vi "ApplyTableBlockAppearance.vi"(5 "Check Mode?":bool, 6 "changed? subarray":bool[][](array[boolean]), 7 "Change start":T1, 8 "error in (no error)":errorcluster, 9 "Mode Index":i32=2, 10 "Col Array in":refnum<class "Column.lvclass">[](array[class]), 11 "Table Ref in":refnum<vi>) -> (0 "error out":errorcluster)   [LabVIEW 2013]
doc: "Selectively format a block-portion of the SetList table based on present value. Since the only* columns whose value changes the formatting are digital (Group is a child), only these are checked. \n*The only exception is the Mode column which is also checked if requested with \"Check Mode?\"."
uses:
  ColumnVIs/Column/Column.lvclass
  <vilib>/Utility/miscctls.llb/LVRowAndColumnTypeDef.ctl
  ColumnVIs/DigitalCol/DigitalCol.lvclass
panel:
  out "Digitals colored":i32
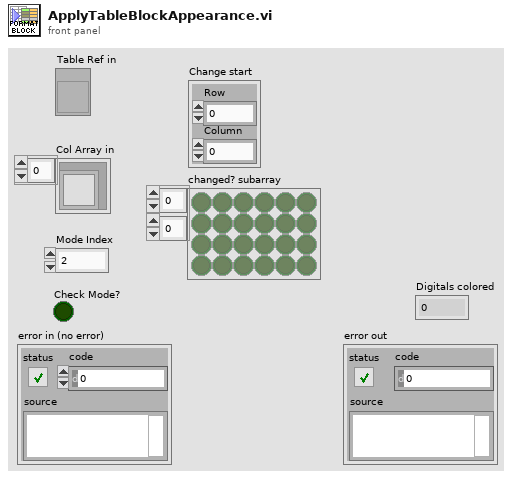
[diagram p1: front panel]
types:
  T1 = typedef "LVRowAndColumnTypeDef.ctl" = cluster{"Row":i32, "Column":i32}
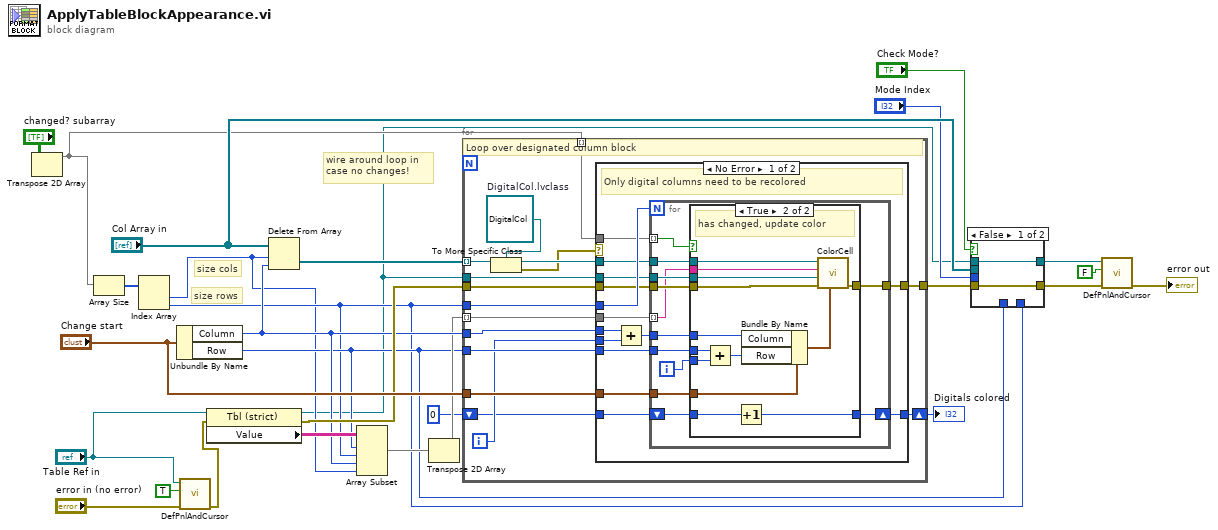
[diagram p0: block diagram]
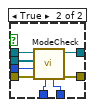
[diagram p2: hidden frame]
diagram:
  # "wire around loop in \ncase no changes!"
  # "size rows"
  # "size cols"
  n1 = Transpose 2D Array(2D array="changed? subarray") -> (transposed array=w4:bool[][])
  n2 = Array Size(array=w4) -> (size(s)=w8:i32[])
  n3 = Index Array(array=w8) -> (element #1=w5:i32, element #2=w6:i32)  [unwired: 2 in]
  n4 = Unbundle By Name("Change start") -> ("Column"=w19:i32, "Row"=w15:i32)
  n5 = call "DefPnlAndCursor.vi"("error in (no error)"="error in (no error)", "DeferPanUpdts?"=TRUE ("Defer Panel Updates"), "Tbl Ctrl Refnum"="Table Ref in") -> ("error out"=w14:errorcluster)  [unwired: 8 in]
  n6 = property class="Tbl (strict)"(reference="Table Ref in", error in=w14) -> (reference out=w1:refnum<vi>, error out=w20:errorcluster, "Value"=w21:string[][])
  n7 = Delete From Array(array="Col Array in", length=w5, index=w19) -> (deleted portion=w24:refnum<class "Column.lvclass">[])  [unwired: 1 out]
  n8 = Array Subset(array=w21, index (row)=w15, length (row)=w6, index (col)=w19, length (col)=w5) -> (w17:string[][])
  n9 = Transpose 2D Array(2D array=w17) -> (transposed array=w16:string[][])
  n10 = for {
    tunnel: w24 -> [w38] mode=indexing
    tunnel: w6 -> [w44]
    tunnel: "Change start" -> [w43]
    tunnel: w15 -> [w42]
    tunnel: w19 -> [w40]
    tunnel: w1 -> [w39]
    tunnel: w20 -> [w34]
    tunnel: [w33] -> w23
    tunnel: w16 -> [w32] mode=indexing
    tunnel: w4 -> [w31] mode=indexing
    shift-right: [w29] -> w2
    shift-left: 0 -> [w30]
    i -> [w41]
    w36 = refnum<class "DigitalCol.lvclass"> refnum  # DigitalCol.lvclass
    # "Loop over designated column block"
    n11 = To More Specific Class(target class=w36, reference=w38) -> (specific class reference=w37:refnum<class "DigitalCol.lvclass">, error out=w35:errorcluster)  [unwired: 1 in]
    n12 = case shown="No Error" w35 {
      tunnel: w44 -> [w58 _]
      tunnel: w43 -> [w57 _]
      tunnel: w42 -> [w56 _]
      tunnel: w41 -> [w54 _]
      tunnel: w40 -> [w53 _]
      tunnel: w39 -> [w52 _]
      tunnel: w37 -> [w51 _]
      tunnel: w34 -> [w50 w87]
      tunnel: [w49 w87] -> w33
      tunnel: w32 -> [w48 _]
      tunnel: w31 -> [w47 _]
      tunnel: w30 -> [w46 w86]
      tunnel: [w45 w86] -> w29
      frame No Error {
        # "Only digital columns need to be recolored"
        n13 = Add(x=w53, y=w54) -> (x+y=w55:i32)
        n14 = for {
          N: w58 -> [_]
          tunnel: w57 -> [w70]
          tunnel: w56 -> [w68]
          tunnel: w55 -> [w67]
          tunnel: w51 -> [w64]
          tunnel: w52 -> [w65]
          tunnel: w50 -> [w66]
          tunnel: [w63] -> w49
          tunnel: w48 -> [w62] mode=indexing
          tunnel: w47 -> [w61] mode=indexing
          shift-right: [w59] -> w45
          shift-left: w46 -> [w60]
          i -> [w69]
          n15 = case shown="True" w61 {
            tunnel: w70 -> [_ w85]
            tunnel: w69 -> [_ w84]
            tunnel: w68 -> [_ w83]
            tunnel: w67 -> [_ w82]
            tunnel: w66 -> [w72 w79]
            tunnel: w65 -> [_ w78]
            tunnel: w64 -> [_ w77]
            tunnel: [w72 w76] -> w63
            tunnel: w62 -> [_ w75]
            tunnel: w60 -> [w71 w74]
            tunnel: [w71 w73] -> w59
            frame False {
              # "no actual change"
            }
            frame True {
              # "has changed, update color"
              n16 = Add(x=w83, y=w84) -> (x+y=w81:i32)
              n17 = Increment(x=w74) -> (x+1=w73:i32)
              n18 = Bundle By Name(cluster=w85, "Column"=w82, "Row"=w81) -> (w80:T1)
              n19 = call-dynamic "ColorCell.vi"("Cell Position"=w80, "error in (no error)"=w79, "Table CtlRef In"=w78, "Value"=w75, "DigitalCol in"=w77) -> ("error out"=w76:errorcluster)  [unwired: 4 in, 2 out]
            }
          }
        }
      }
      frame Error {
        # "No need to check coloring!"
      }
    }
  }
  "Digitals colored" <- w2
  n20 = case shown="False" "Check Mode?" {
    tunnel: w23 -> [w89 w97]
    tunnel: "Mode Index" -> [_ w96]
    tunnel: "Col Array in" -> [_ w95]
    tunnel: [w89 w94] -> w11
    tunnel: w1 -> [w88 w93]
    tunnel: w15 -> [_ w92]
    tunnel: w6 -> [_ w91]
    tunnel: [w88 w90] -> w12
    frame False {
    }
    frame True {
      n21 = call "ModeCheck.vi"("Row Span (all)"=w91, "Start Row (first, DISAB only)"=w92, "error in (no error)"=w97, "mode col. index"=w96, "Col Array in"=w95, "Table Ref in"=w93) -> ("error out"=w94:errorcluster, "Table Ref out"=w90:refnum<vi>)  [unwired: 4 in]
    }
  }
  n22 = call "DefPnlAndCursor.vi"("error in (no error)"=w11, "DeferPanUpdts?"=FALSE, "Tbl Ctrl Refnum"=w12) -> ("error out"=→"error out":errorcluster)  [unwired: 8 in]
